vi "Car-ultrasonic-poc.vi"() -> ()   [LabVIEW 2026]
uses:
  CTI-Grove/Examples/Sourcecode/cti-drivers-lv-visa-simple/Examples/Driver/Public/Digital Direction.ctl
  CTI-Grove/Examples/Sourcecode/cti-drivers-lv-visa-simple/Examples/Driver/CTIPicoVISA.lvlib
panel:
  out "Waveform Chart":dbl(graph)
  out "Numeric 2":i32
  in  "Numeric":i32
  out "Identity":T1
  in  "stop":bool
  in  "VISA resource name in":refnum<visa-resource-name>="ASRL1::INSTR"
  out "error out":errorcluster
  # "https://wiki.seeedstudio.com/Grove-Passive-Buzzer/"
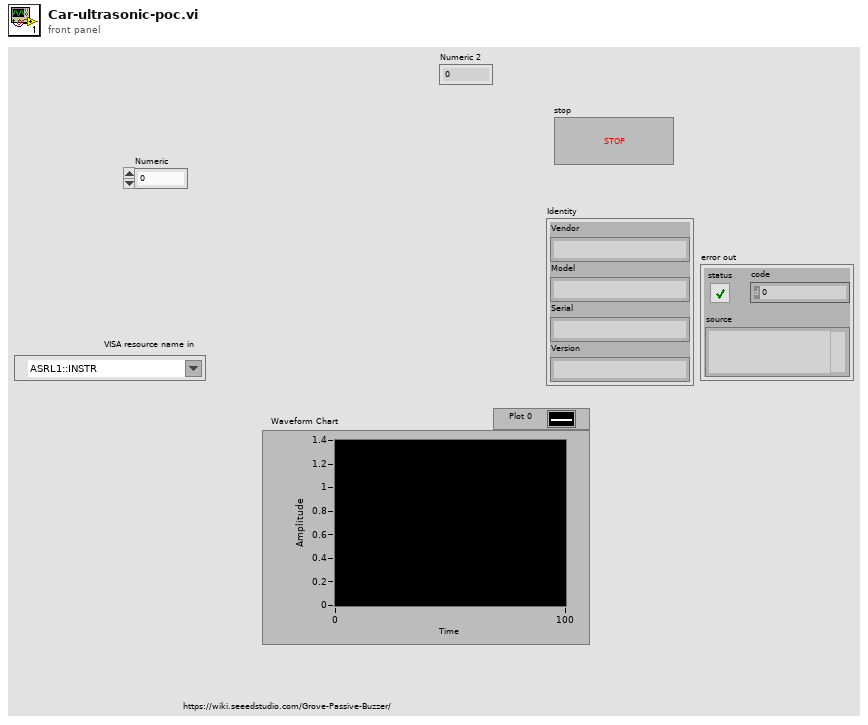
[diagram p1: front panel]
types:
  T1 = cluster{"Vendor":string, "Model":string, "Serial":string, "Version":string}
  T2 = typedef "CTIPicoVISA.lvlib/Digital Direction.ctl" = enum16{"In", "Out"}
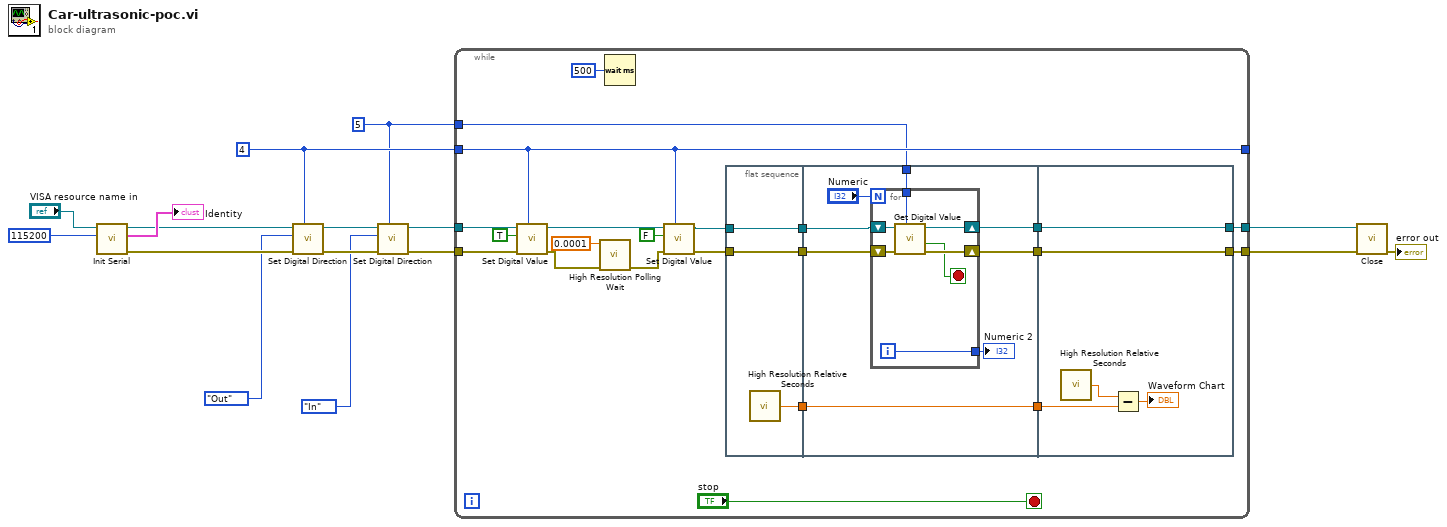
[diagram p0: block diagram]
diagram:
  w3 = 5 ("GPIO")
  w10 = 4 ("GPIO")
  n1 = call "Init Serial.vi"("Baud (115200)"=u32 115200, "VISA resource name in"="VISA resource name in") -> ("error out"=w11:errorcluster, "Identity"=→"Identity":T1, "VISA resource name Out"=w12:refnum<visa-resource-name>)  [unwired: 7 in]
  n2 = call "Set Digital Direction.vi"("GPIO"=w10, "error in (no error)"=w11, "Direction"=Digital_Direction."Out", "VISA resource name in"=w12) -> ("error out"=w7:errorcluster, "VISA resource name"=w8:refnum<visa-resource-name>)  [unwired: 6 in]
  n3 = call "Set Digital Direction.vi"("GPIO"=w3, "error in (no error)"=w7, "Direction"=Digital_Direction."In", "VISA resource name in"=w8) -> ("error out"=w4:errorcluster, "VISA resource name"=w5:refnum<visa-resource-name>)  [unwired: 6 in]
  n4 = while {
    tunnel: w10 -> [w26]
    tunnel: [w26] -> _
    tunnel: w5 -> [w36]
    tunnel: w4 -> [w35]
    tunnel: w3 -> [w25]
    tunnel: [w19] -> w2
    tunnel: [w18] -> w1
    stop <- "stop" stop-if-true
    n5 = call "Set Digital Value.vi"("GPIO"=w26, "error in (no error)"=w35, "Value"=TRUE, "VISA resource name in"=w36) -> ("error out"=w32:errorcluster, "VISA resource name"=w30:refnum<visa-resource-name>)  [unwired: 6 in]
    n6 = call <vilib>:"High Resolution Polling Wait.vi"("error in (no error)"=w32, "seconds to wait"=0.0001) -> ("error out"=w29:errorcluster)  [unwired: 9 in]
    n7 = Wait (ms)(milliseconds to wait=u32 500) -> ()  [unwired: 1 out]
    n8 = call "Set Digital Value.vi"("GPIO"=w26, "error in (no error)"=w29, "Value"=FALSE, "VISA resource name in"=w30) -> ("error out"=w27:errorcluster, "VISA resource name"=w28:refnum<visa-resource-name>)  [unwired: 6 in]
    n9 = flat-sequence {
      tunnel: w27 -> [w40]
      tunnel: w28 -> [w41]
      tunnel: [w41] -> w24
      tunnel: [w40] -> w23
      tunnel: [w39] -> w22
      tunnel: w25 -> [w47]
      tunnel: w24 -> [w49]
      tunnel: w23 -> [w48]
      tunnel: w22 -> [w44]
      tunnel: [w44] -> w21
      tunnel: [w43] -> w20
      tunnel: [w42] -> w17
      tunnel: w21 -> [w60]
      tunnel: w20 -> [w59]
      tunnel: [w59] -> w19
      tunnel: [w58] -> w18
      tunnel: w17 -> [w58]
      frame #0 {
        n10 = call <vilib>:"High Resolution Relative Seconds.vi"() -> ("relative seconds"=w39:dbl)
      }
      frame #1 {
        n11 = for {
          N: "Numeric" -> [_]
          tunnel: w47 -> [w52]
          shift-right: [w55] -> w42
          shift-left: w48 -> [w56]
          shift-right: [w53] -> w43
          shift-left: w49 -> [w54]
          tunnel: [w50] -> w45
          i -> [w50]
          stop <- w51 stop-if-true
          n12 = call "Get Digital Value.vi"("GPIO"=w52, "error in (no error)"=w56, "VISA resource name in"=w54) -> ("error out"=w55:errorcluster, "Value"=w51:bool, "VISA resource name"=w53:refnum<visa-resource-name>)  [unwired: 6 in]
        }
        "Numeric 2" <- w45
      }
      frame #2 {
        n13 = call <vilib>:"High Resolution Relative Seconds.vi"() -> ("relative seconds"=w61:dbl)
        n14 = Subtract(x=w61, y=w60) -> (x-y=→"Waveform Chart":dbl)
      }
    }
  }
  n15 = call "Close.vi"("error in (no error)"=w1, "VISA resource name in"=w2) -> ("error out"=→"error out":errorcluster)  [unwired: 9 in]
